vi "Dialog_Arrow Up on Listbox.vi"(10 "String Ref":refnum<vi>, 11 "TreeControl in":refnum<vi>) -> (3 "discard":bool)   [LabVIEW 2023]
doc: "If one item is selected and it's the last item, and the down arrow is pressed, move to first item in listbox"
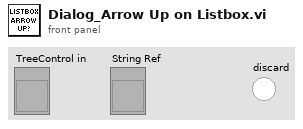
[diagram p1: front panel]
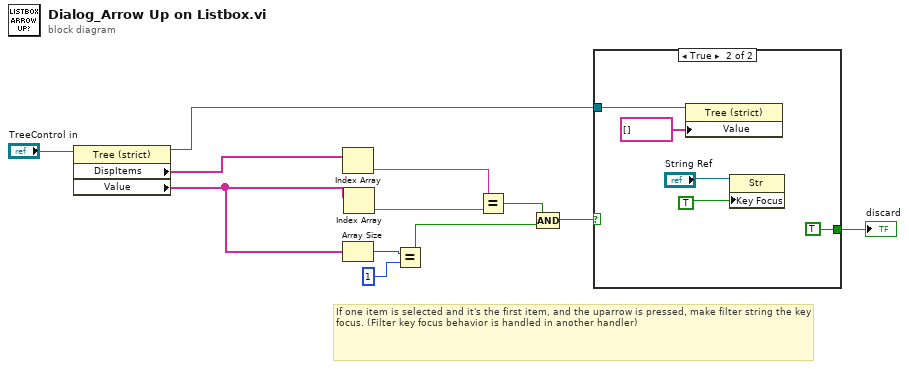
[diagram p0: block diagram]
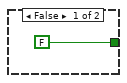
[diagram p2: hidden frame]
diagram:
  # "If one item is selected and it's the first item, and the uparrow is pressed, make filter string the key focus. (Filter key focus behavior is handled in another handler)"
  n1 = property class="Tree (strict)"(reference="TreeControl in") -> (reference out=w1:refnum<vi>, "DispItems"=w12:string[], "Value"=w8:string[])  [unwired: 1 in, 1 out]
  n2 = Index Array(array=w12) -> (element=w2:string)  [unwired: 1 in]
  n3 = Array Size(array=w8) -> (size(s)=w10:i32)
  n4 = Index Array(array=w8) -> (element=w7:string)  [unwired: 1 in]
  n5 = Equal?(x=w10, y=1) -> (x = y?=w5:bool)
  n6 = Equal?(x=w2, y=w7) -> (x = y?=w6:bool)
  n7 = Compound Arithmetic op=AND(w6, w5) -> (w4:bool)
  n8 = case shown="True" w4 {
    tunnel: [FALSE ("discard") TRUE ("discard")] -> w3
    tunnel: w1 -> [_ w14]
    frame False {
    }
    frame True {
      n9 = property class="Tree (strict)"(reference=w14, "Value"=string[] []) -> ()  [unwired: 1 in, 2 out]
      n10 = property class="Str"(reference="String Ref", "Key Focus"=TRUE) -> ()  [unwired: 1 in, 2 out]
    }
  }
  "discard" <- w3
